vi "Cosim.vi"() -> ()   [LabVIEW 2015]
uses:
  <vilib>/Simulation/Scripting/Companion Diagram/SimConfigNode/SimParams.ctl
  <vilib>/Simulation/Scripting/Companion Diagram/SimConfigNode/_simSolvers.ctl
  <vilib>/Simulation/Implementation/Shared/SIMSCR Execution Mode.ctl
  <vilib>/Simulation/Param Hierarchy/Typedefs/SIMPH Param Control Actions.ctl
  SPWM/Signal.ctl
  <vilib>/Simulation/Implementation/Shared/NILVSim_ParamChanged.vi
  <vilib>/Simulation/Implementation/Shared/NILVSIM_BeginStep.vi
  <vilib>/Simulation/DataSources/Implementation/NILVSim Sine Wave.llb/SIM Sine Wave (scalar).vi
  <vilib>/Simulation/Implementation/Shared/NILVSim_Manager.vi
  <vilib>/Utility/error.llb/Clear Errors.vi
  <vilib>/Simulation/Implementation/Shared/NILVSim_FinalizeModel.vi
  <vilib>/Simulation/Implementation/Shared/SIM Unbundle Sim Info.vi
  <vilib>/Simulation/Implementation/Shared/NILVSim_Initialize.vi
  <vilib>/Simulation/Utility/Implementation/NILVSim Get Time and IsAcceptedStep.vi
  SPWM/Core.vi
  <vilib>/Simulation/Implementation/Shared/SIMSH Read Queue.vi
  <vilib>/Simulation/Implementation/Shared/NILVSim_GetModelError.vi
  <vilib>/Simulation/Implementation/Shared/SIM Bundle Sim Info.vi
  <vilib>/Simulation/Scripting/Companion Diagram/SimConfigNode/SimDog.xnode
  <vilib>/Simulation/Implementation/XNodeFramework/SimXNode/SimX.xnode
  <vilib>/Simulation/EMI/Plugins/Multisim Design/MultisimEMICtrl.dll
  SPWMInterface/SPWMInterface.lvlib
  SPWM/SPWM.lvlib
  <vilib>/Simulation/Implementation/Shared/NI_SIM_Implementation.lvlib
panel:
  out "x/y":dbl[][](graph)
  in  "frequency":dbl=0.5
  in  "amplitude":dbl=1.0
  in  "enable":bool
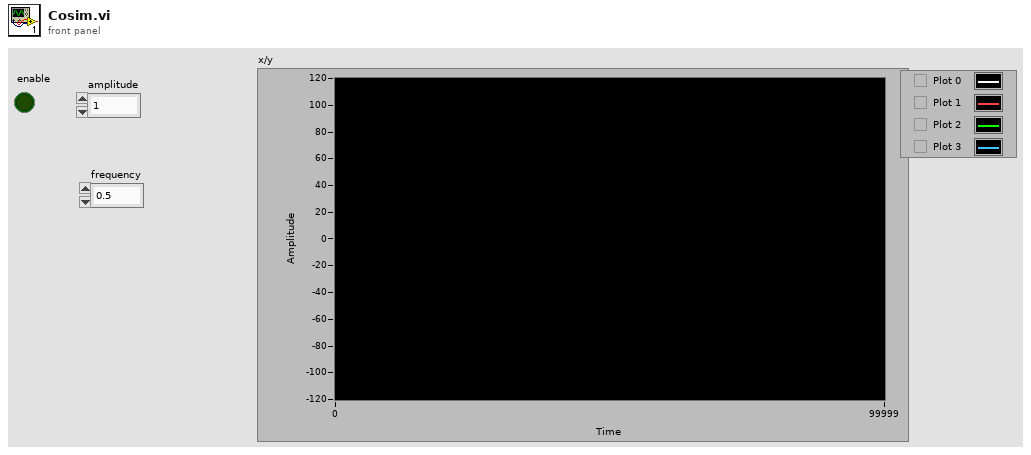
[diagram p1: front panel]
types:
  T1 = typedef "SPWM.lvlib/SwitchConfig.ctl" = cluster{"FreqCarrier":u32, "DeadtimeTicks":u8, "TriangleInc":fxp<+/-,32,4>}
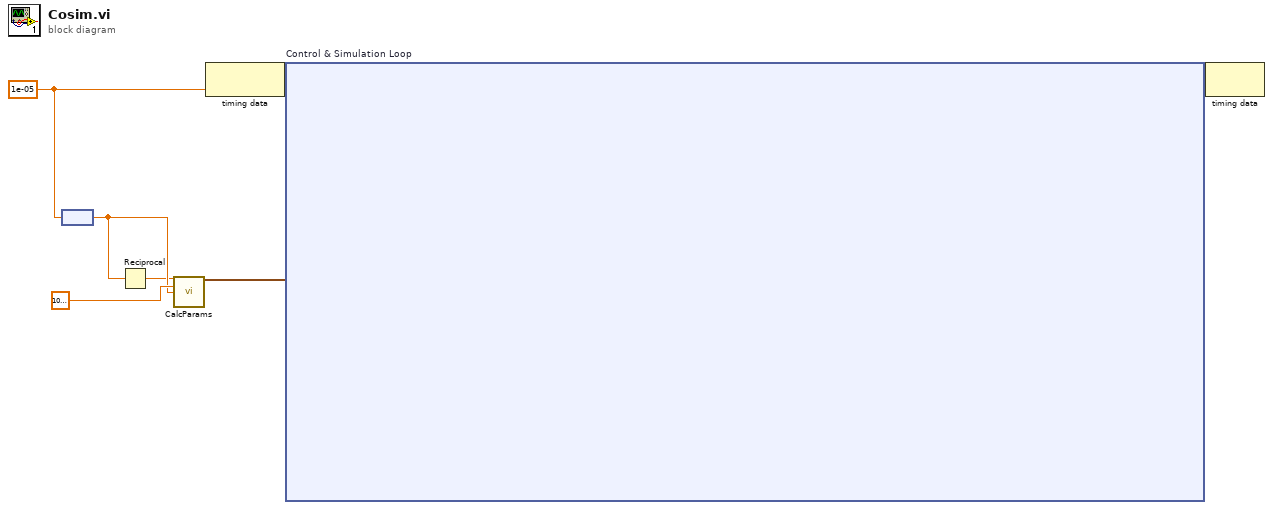
[diagram p0: block diagram]
diagram:
  w3 = 1e-05 ("Step Size (s)")
  n1 = node(w3) -> (w2:dbl[unit])
  n2 = Reciprocal(x=w2) -> (1/x=w1:dbl[unit])
  n3 = call "CalcParams.vi"("ClkRate"=w1, "fc"=dbl[unit] 10000.0, "Deadtime"=w2) -> ("Parameters"=w5:T1)  [unwired: 12 in]
  n4 = node-c288(w3) -> (w7:variant)
  n5 = node-c254 "Control & Simulation Loop"(w7, w5) -> (w6:variant)
  n6 = node-c288(w6) -> ()  [unwired: 1 out]
